vi "Periodic Tasks.vi"(7 "Chassis X SPD":dbl=0.65, 8 "error in":errorcluster) -> ()   [LabVIEW 2019]
doc: "This VI runs in parallel to other tasks. It can contain as many user-defined periodic loops as you need. These can carry out PID or other sorts of timed response."
uses:
  <vilib>/Rock Robotics/WPI/Utilities/WPI_GetSetVariantRefNum.vi
  Robot Global Data.vi
  <vilib>/Rock Robotics/Network Tables/NT Read Number.vi
  <vilib>/Rock Robotics/Network Tables/NT Write Number.vi
  <vilib>/Rock Robotics/WPI/RobotDrive/WPI_RobotDriveArcadeDrive_Standard(NoSaturation).vi
  <vilib>/Rock Robotics/Network Tables/NT Read Boolean.vi
panel:
  out "Bottom RPM":dbl
  out "Top RPM":dbl
  out "Offset Y":dbl
  out "Offset X":dbl
  in  "h1":dbl
  in  "a1":dbl=35.0
  in  "Chassis Y SPD":dbl=0.65
  # "The tilt applied to the Limelight when mounted"
  # "Height of the floor to the center of the limelight"
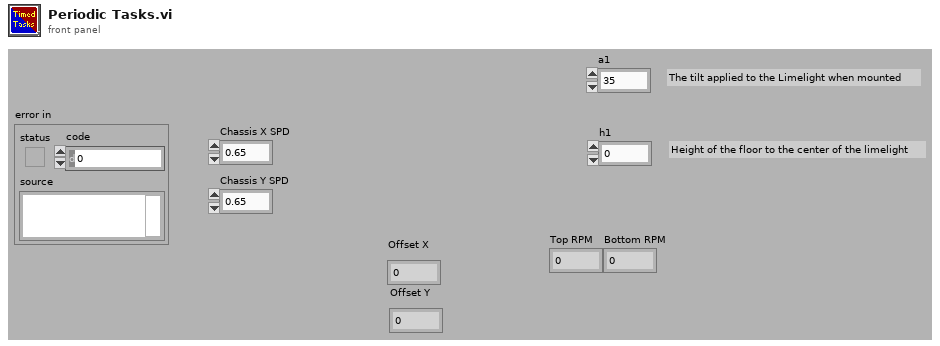
[diagram p1: front panel]
types:
  T1 = typedef "WPI_JoystickDevRef.ctl" = cluster{"Device":T2}
  T2 = typedef "WPI_JoystickDeviceEnum.ctl" = enum16{"USB 0", "USB 1", "USB 2", "USB 3", "USB 4", "USB 5"}
  T3 = typedef "WPI_RobotDriveDevRef.ctl" = cluster{"DevStatus":errorcluster, "Motors[]":T4[], "Square Inputs":bool, "Max Output":dbl}
  T4 = typedef "WPI_MotorControlDeviceRef.ctl" = cluster{"DeviceStatus":errorcluster, "Type":T5, "PWM":cluster{"PWM Channel":T6, "DeadBand":T7}, "CAN":cluster{"Device Number":u8, "SetOutput VI Ref":variant, "GetOutput VI Ref":variant, "Enable VI Ref":variant, "Disable VI Ref":variant, "Data":variant}, "Invert":bool, "DIO PWM":cluster{"PWM \"Enable\" Channel":T6, "DIOChannel":T8, "PWM Rate":dbl}}
  T5 = typedef "WPI_MotorControlType.ctl" = enum16{"PWM", "CAN", "DIO PWM"}
  T6 = typedef "FPGA_DIOPWMChannel.ctl" = enum8{"PWM 0", "PWM 1", "PWM 2", "PWM 3", "PWM 4", "PWM 5", "PWM 6", "PWM 7", "PWM 8", "PWM 9", "PWM MXP 0", "PWM MXP 1", "PWM MXP 2", "PWM MXP 3", "PWM MXP 4", "PWM MXP 5", "PWM MXP 6", "PWM MXP 7", "PWM MXP 8", "PWM MXP 9", "Invalid"}
  T7 = typedef "WPI_PWMDeadband.ctl" = cluster{"Name":string, "maxPositivePwm":i32, "minPositivePwm":i32, "centerPwm":i32, "maxNegativePwm":i32, "minNegativePwm":i32, "angularRange":u16}
  T8 = typedef "FPGA_DIOChannel.ctl" = enum8{"DIO 0", "DIO 1", "DIO 2", "DIO 3", "DIO 4", "DIO 5", "DIO 6", "DIO 7", "DIO 8", "DIO 9", "DIO MXP 0", "DIO MXP 1", "DIO MXP 2", "DIO MXP 3", "DIO MXP 4", "DIO MXP 5", "DIO MXP 6", "DIO MXP 7", "DIO MXP 8", "DIO MXP 9", "DIO MXP 10", "DIO MXP 11", "DIO MXP 12", "DIO MXP 13", "DIO MXP 14", "DIO MXP 15", "SPI Port CS1", "SPI Port CS2", "SPI Port CS3", "SPI Port MISO", "SPI Port MOSI", "Invalid"}
  T9 = cluster{"JoystickDevRef":T1, "RobotDriveDevRef":T3}
  T10 = typedef "WPI_ServoDeviceRef.ctl" = cluster{"DeviceStatus":errorcluster, "PWM Channel":T6, "DeadBand":T7}
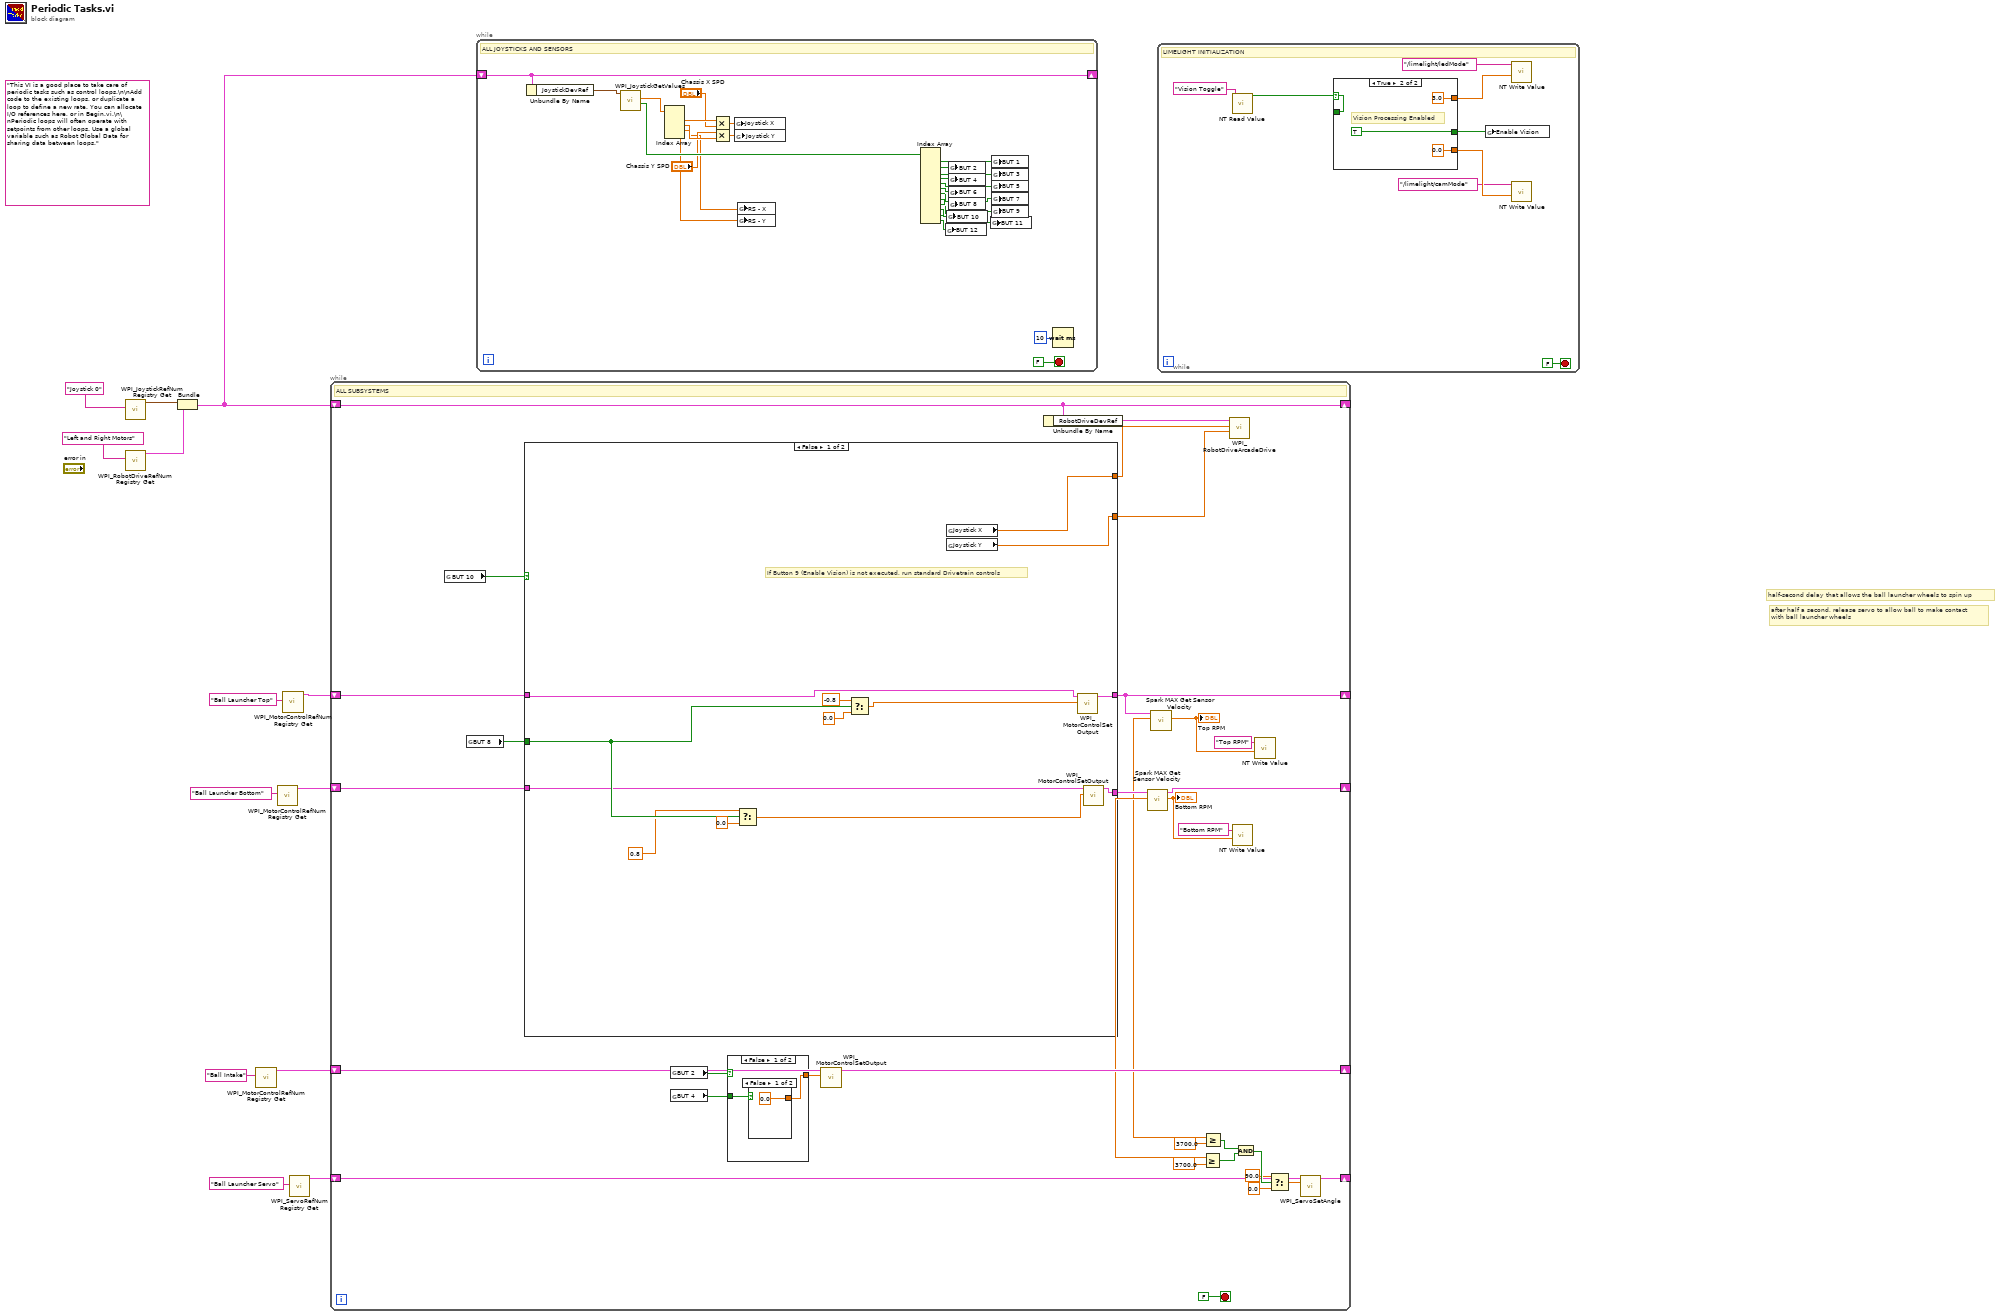
[diagram p0: block diagram]
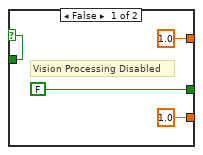
[diagram p2: hidden frame]
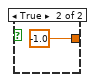
[diagram p3: hidden frame]
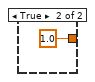
[diagram p4: hidden frame]
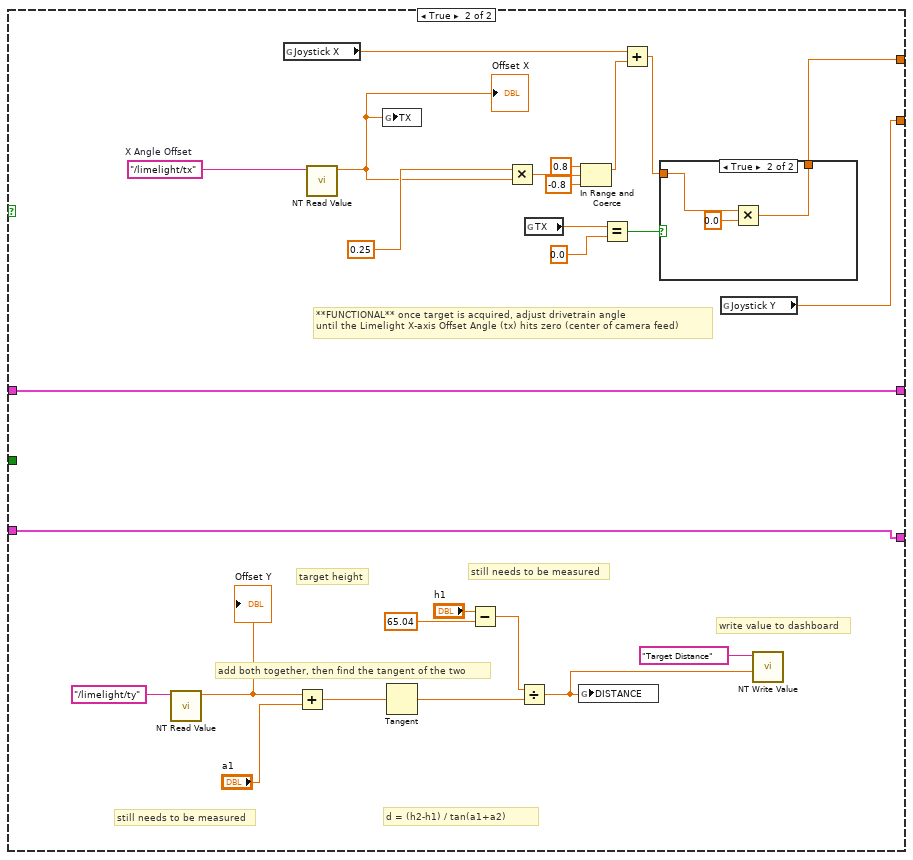
[diagram p5: hidden frame]
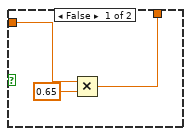
[diagram p6: hidden frame]
diagram:
  (unwired) "This VI is a good place to take care of periodic tasks such as control loops.\n\nAdd code to the existing loops, or duplicate a loop to define a new rate. You can allocate I/O references here, or in Begin.vi.\n\nPeriodic loops will often operate with setpoints from other loops. Use a global variable such as Robot Global Data for sharing data between loops."
  # "after half a second, release servo to allow ball to make contact\nwith ball launcher wheels"
  # "half-second delay that allows the ball launcher wheels to spin up"
  n1 = call <vilib>:"WPI_JoystickRefNum Registry Get.vi"("refnum name"="Joystick 0") -> ("JoystickDevRef"=w11:T1)  [unwired: 1 in, 9 out]
  n2 = call <vilib>:"WPI_RobotDriveRefNum Registry Get.vi"("refnum name"="Left and Right Motors") -> ("RobotDriveDevRef"=w10:T3)  [unwired: 1 in, 9 out]
  n3 = Bundle("JoystickDevRef"=w11, "RobotDriveDevRef"=w10) -> (w9:T9)  [unwired: 1 out]
  n4 = call <vilib>:"WPI_MotorControlRefNum Registry Get.vi"("refnum name"="Ball Intake") -> ("MotorControlDevRef"=w6:T4)  [unwired: 9 in, 1 out]
  n5 = call <vilib>:"WPI_MotorControlRefNum Registry Get.vi"("refnum name"="Ball Launcher Bottom") -> ("MotorControlDevRef"=w3:T4)  [unwired: 9 in, 1 out]
  n6 = call <vilib>:"WPI_MotorControlRefNum Registry Get.vi"("refnum name"="Ball Launcher Top") -> ("MotorControlDevRef"=w8:T4)  [unwired: 9 in, 1 out]
  n7 = call <vilib>:"WPI_ServoRefNum Registry Get.vi"("refnum name"="Ball Launcher Servo") -> ("ServoDeviceRef"=w2:T10)  [unwired: 9 in, 1 out]
  n8 = while {
    shift-right: [w43] -> _
    shift-left: w9 -> [w43]
    shift-right: [w31] -> _
    shift-left: w8 -> [w37]
    shift-right: [w33] -> _
    shift-left: w6 -> [w32]
    shift-right: [w28] -> _
    shift-left: w3 -> [w30]
    shift-right: [w27] -> _
    shift-left: w2 -> [w18]
    stop <- FALSE stop-if-true
    # "ALL SUBSYSTEMS"
    n9 = global read "Robot Global Data.vi" "BUT 10"() -> (w42:bool)
    n10 = global read "Robot Global Data.vi" "BUT 8"() -> (w38:bool)
    n11 = case shown="False" w42 {
      tunnel: [w62 w80] -> w40
      tunnel: [w61 w76] -> w39
      tunnel: w38 -> [w55 _]
      tunnel: w37 -> [w57 w65]
      tunnel: [w58 w65] -> w31
      tunnel: w30 -> [w52 w63]
      tunnel: [w50 w63] -> w29
      frame False {
        # "If Button 9 (Enable Vision) is not executed, run standard Drivetrain controls"
        n12 = Select(t=0.8, s=w55, f=0.0) -> (s? t:f=w51:dbl)
        n13 = Select(t=-0.8, s=w55, f=0.0) -> (s? t:f=w56:dbl)
        n14 = global read "Robot Global Data.vi" "Joystick X"() -> (w62:dbl)
        n15 = global read "Robot Global Data.vi" "Joystick Y"() -> (w61:dbl)
        n16 = call <vilib>:"WPI_MotorControlSetOutput.vi"("Output"=w56, "MotorControlDevRef"=w57) -> ("MotorControlDevRef"=w58:T4)  [unwired: 7 in, 2 out]
        n17 = call <vilib>:"WPI_MotorControlSetOutput.vi"("Output"=w51, "MotorControlDevRef"=w52) -> ("MotorControlDevRef"=w50:T4)  [unwired: 7 in, 2 out]
      }
      frame True {
        w88 = "/limelight/tx"  # X Angle Offset
        # "write value to dashboard"
        # "still needs to be measured"
        # "target height"
        # "add both together, then find the tangent of the two"
        # "still needs to be measured"
        # "d = (h2-h1) / tan(a1+a2)"
        # "**FUNCTIONAL** once target is acquired, adjust drivetrain angle \nuntil the Limelight X-axis Offset Angle (tx) hits zero (center of camera feed)"
        n18 = call-poly <vilib>:"NT Read Value.vi"("Name"="/limelight/ty") -> ("Numeric"=w74:dbl)  [unwired: 9 in, 1 out]
        "Offset Y" <- w74
        n19 = global read "Robot Global Data.vi" "Joystick X"() -> (w87:dbl)
        n20 = Add(x=w74, y="a1") -> (x+y=w72:dbl)
        n21 = call-poly <vilib>:"NT Read Value.vi"("Name"=w88) -> ("Numeric"=w64:dbl)  [unwired: 9 in, 1 out]
        "Offset X" <- w64
        n22 = global write "Robot Global Data.vi" "TX"(w64) -> ()
        n23 = Tangent(1:w72) -> (0:w71:dbl)
        n24 = Subtract(x="h1", y=65.04) -> (x-y=w69:dbl)
        n25 = Multiply(x=0.25 ("y"), y=w64) -> (x*y=w85:dbl)
        n26 = Divide(x=w69, y=w71) -> (x/y=w66:dbl)
        n27 = global read "Robot Global Data.vi" "TX"() -> (w78:dbl)
        n28 = global write "Robot Global Data.vi" "DISTANCE"(w66) -> ()
        n29 = In Range and Coerce(upper limit=0.8, x=w85, lower limit=-0.8) -> (coerced(x)=w86:dbl)  [unwired: 1 out]
        n30 = Equal?(x=w78, y=0.0) -> (x = y?=w79:bool)
        n31 = Add(x=w87, y=w86) -> (x+y=w81:dbl)
        n32 = case shown="True" w79 {
          tunnel: w81 -> [w90 w94]
          tunnel: [w91 w92] -> w80
          frame False {
            n33 = Multiply(x=w90, y=0.65) -> (x*y=w91:dbl)
          }
          frame True {
            n34 = Multiply(x=w94, y=0.0) -> (x*y=w92:dbl)
          }
        }
        n35 = global read "Robot Global Data.vi" "Joystick Y"() -> (w76:dbl)
        n36 = call-poly <vilib>:"NT Write Value.vi"("Numeric"=w66, "Name"="Target Distance") -> ()  [unwired: 9 in, 1 out]
      }
    }
    n37 = global read "Robot Global Data.vi" "BUT 2"() -> (w35:bool)
    n38 = global read "Robot Global Data.vi" "BUT 4"() -> (w36:bool)
    n39 = case shown="False" w35 {
      tunnel: [w46 1.0 ("Output")] -> w34
      tunnel: w36 -> [w45 _]
      frame False {
        n40 = case shown="False" w45 {
          tunnel: [0.0 ("Output") -1.0 ("Output")] -> w46
          frame False {
          }
          frame True {
          }
        }
      }
      frame True {
      }
    }
    n41 = call <vilib>:"WPI_MotorControlSetOutput.vi"("Output"=w34, "MotorControlDevRef"=w32) -> ("MotorControlDevRef"=w33:T4)  [unwired: 7 in, 2 out]
    n42 = Unbundle By Name(w43) -> ("RobotDriveDevRef"=w41:T3)
    n43 = call <vilib>:"Spark MAX Get Sensor Velocity.vi"("MotorControlDevRef in"=w29) -> ("Sensor Velocity"=w17:dbl, "MotorControlDevRef out"=w28:T4)  [unwired: 7 in, 2 out]
    "Bottom RPM" <- w17
    n44 = call <vilib>:"Spark MAX Get Sensor Velocity.vi"("MotorControlDevRef in"=w31) -> ("Sensor Velocity"=w14:dbl)  [unwired: 7 in, 3 out]
    "Top RPM" <- w14
    n45 = Greater Or Equal?(x=w17, y=3700.0) -> (x >= y?=w24:bool)
    n46 = Greater Or Equal?(x=w14, y=3700.0) -> (x >= y?=w23:bool)
    n47 = call-poly <vilib>:"WPI_RobotDriveArcadeDrive.vi"("Y axis value"=w39, "X axis value"=w40, "RobotDriveDevRef"=w41) -> ()  [unwired: 6 in, 3 out]
    n48 = call-poly <vilib>:"NT Write Value.vi"("Numeric"=w17, "Name"="Bottom RPM") -> ()  [unwired: 9 in, 1 out]
    n49 = And(x=w23, y=w24) -> (x .and. y?=w21:bool)
    n50 = call-poly <vilib>:"NT Write Value.vi"("Numeric"=w14, "Name"="Top RPM") -> ()  [unwired: 9 in, 1 out]
    n51 = Select(t=90.0, s=w21, f=0.0) -> (s? t:f=w22:dbl)
    n52 = call <vilib>:"WPI_ServoSetAngle.vi"("Angle"=w22, "ServoDeviceRef"=w18) -> ("ServoDeviceRef"=w27:T10)  [unwired: 8 in, 1 out]
  }
  n53 = while {
    shift-right: [w104] -> _
    shift-left: w9 -> [w104]
    stop <- FALSE stop-if-true
    # "ALL JOYSTICKS AND SENSORS"
    n54 = Unbundle By Name(w104) -> ("JoystickDevRef"=w118:T1)
    n55 = call <vilib>:"WPI_JoystickGetValues.vi"("JoystickDevRef"=w118) -> ("Buttons"=w117:bool[], "Axes"=w103:dbl[])  [unwired: 6 in, 3 out]
    n56 = Index Array(array=w103) -> (element #1=w100:dbl, element #2=w99:dbl, element #3=w96:dbl, element #4=w95:dbl)  [unwired: 4 in]
    n57 = Multiply(x=w100, y="Chassis X SPD") -> (x*y=w102:dbl)
    n58 = Multiply(x="Chassis Y SPD", y=w99) -> (x*y=w101:dbl)
    n59 = global write "Robot Global Data.vi" "Joystick X"(w102) -> ()
    n60 = global write "Robot Global Data.vi" "Joystick Y"(w101) -> ()
    n61 = global write "Robot Global Data.vi" "RS - X"(w96) -> ()
    n62 = global write "Robot Global Data.vi" "RS - Y"(w95) -> ()
    n63 = Index Array(array=w117) -> (element #1=w116:bool, element #2=w115:bool, element #3=w114:bool, element #4=w113:bool, element #5=w112:bool, element #6=w111:bool, element #7=w110:bool, element #8=w109:bool, element #9=w108:bool, element #10=w107:bool, element #11=w106:bool, element #12=w105:bool)  [unwired: 12 in]
    n64 = global write "Robot Global Data.vi" "BUT 12"(w105) -> ()
    n65 = global write "Robot Global Data.vi" "BUT 10"(w107) -> ()
    n66 = global write "Robot Global Data.vi" "BUT 2"(w115) -> ()
    n67 = global write "Robot Global Data.vi" "BUT 4"(w113) -> ()
    n68 = global write "Robot Global Data.vi" "BUT 6"(w111) -> ()
    n69 = global write "Robot Global Data.vi" "BUT 8"(w109) -> ()
    n70 = global write "Robot Global Data.vi" "BUT 11"(w106) -> ()
    n71 = global write "Robot Global Data.vi" "BUT 1"(w116) -> ()
    n72 = global write "Robot Global Data.vi" "BUT 3"(w114) -> ()
    n73 = global write "Robot Global Data.vi" "BUT 5"(w112) -> ()
    n74 = global write "Robot Global Data.vi" "BUT 7"(w110) -> ()
    n75 = global write "Robot Global Data.vi" "BUT 9"(w108) -> ()
    n76 = Wait (ms)(milliseconds to wait=u32 10) -> ()  [unwired: 1 out]
  }
  n77 = while {
    stop <- FALSE stop-if-true
    # "LIMELIGHT INITIALIZATION"
    n78 = call-poly <vilib>:"NT Read Value.vi"("Name"="Vision Toggle") -> ("Boolean"=w122:bool)  [unwired: 9 in, 1 out]
    n79 = case shown="True" w122 {
      selector: w122 -> [w129 w133]
      tunnel: [FALSE ("Enable Vision") TRUE ("Enable Vision")] -> w126
      tunnel: [1.0 ("Numeric") 0.0 ("Numeric")] -> w127
      tunnel: [1.0 ("Numeric") 3.0 ("Numeric")] -> w128
      tunnel: [w129 w133] -> _
      frame False {
        # "Vision Processing Disabled"
      }
      frame True {
        # "Vision Processing Enabled"
      }
    }
    n80 = global write "Robot Global Data.vi" "Enable Vision"(w126) -> ()
    n81 = call-poly <vilib>:"NT Write Value.vi"("Numeric"=w128, "Name"="/limelight/ledMode") -> ()  [unwired: 9 in, 1 out]
    n82 = call-poly <vilib>:"NT Write Value.vi"("Numeric"=w127, "Name"="/limelight/camMode") -> ()  [unwired: 9 in, 1 out]
  }
